vi "Write TrigPulsWidthMin(ticks).vi"(8 "error in (no error)":errorcluster, 10 "TrigPulsWidthMin(ticks)":u64, 11 "TrigBoxINIFileClass in":refnum<class "TrigBoxINIFileClass.lvclass">) -> (0 "error out":errorcluster, 3 "TrigBoxINIFileClass out":refnum<class "TrigBoxINIFileClass.lvclass">)   [LabVIEW 2013, in "TrigBoxINIFileClass.lvclass"]
uses:
  TrigBoxINIFileClass.lvclass
  TrigBoxINIFileClass.lvclass/TrigBoxINIFileClass.ctl
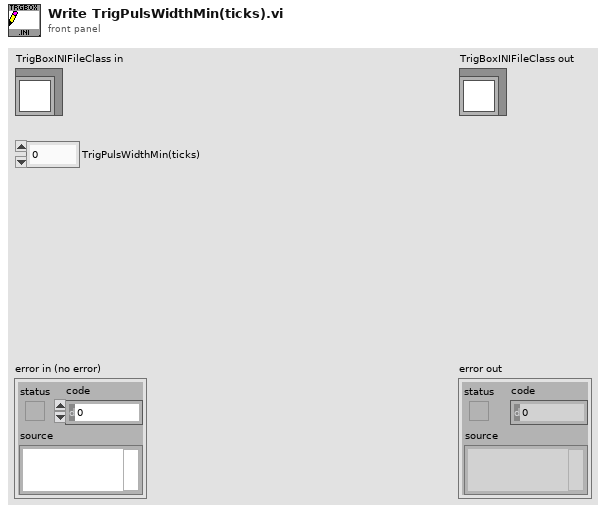
[diagram p1: front panel]
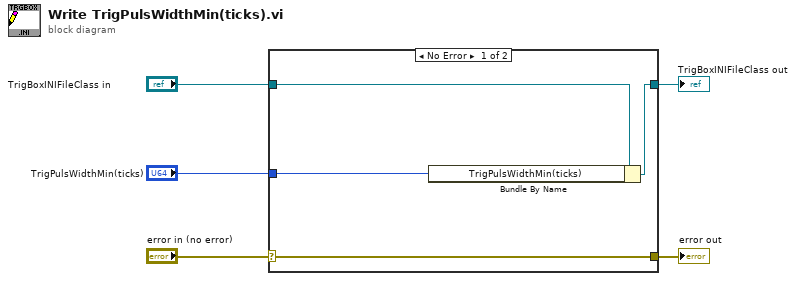
[diagram p0: block diagram]
diagram:
  n1 = case shown="No Error" "error in (no error)" {
    selector: "error in (no error)" -> [w9 w10]
    tunnel: [w9 w10] -> w4
    tunnel: [w7 w11] -> w2
    tunnel: "TrigBoxINIFileClass in" -> [w8 w11]
    tunnel: "TrigPulsWidthMin(ticks)" -> [w6 _]
    frame No Error {
      n2 = Bundle By Name(cluster=w8, "TrigPulsWidthMin(ticks)"=w6) -> (w7:refnum<class "TrigBoxINIFileClass.lvclass">)
    }
    frame Error {
    }
  }
  "error out" <- w4
  "TrigBoxINIFileClass out" <- w2
